vi "Get Fit Length.vi"(8 "error in (no error)":errorcluster, 11 "Abstract Fit in":refnum<class "Abstract Fit.lvclass">) -> (0 "error out":errorcluster, 2 "Length":i32, 3 "Abstract Fit out":refnum<class "Abstract Fit.lvclass">)   [LabVIEW 2016, in "Abstract Fit.lvclass"]
uses:
  Abstract Fit.lvclass
  Abstract Fit.lvclass/Abstract Fit.ctl
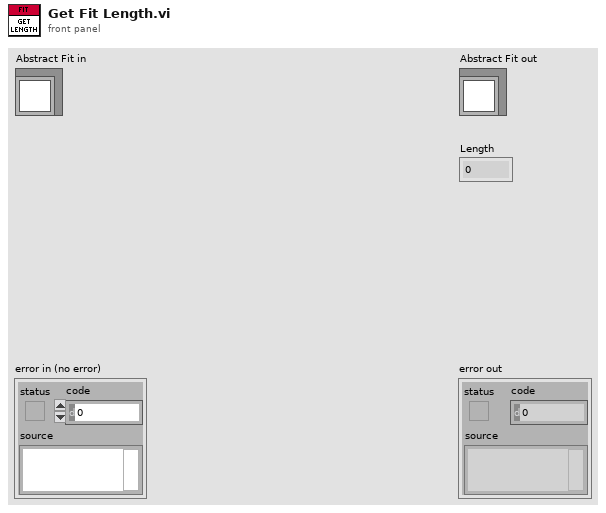
[diagram p1: front panel]
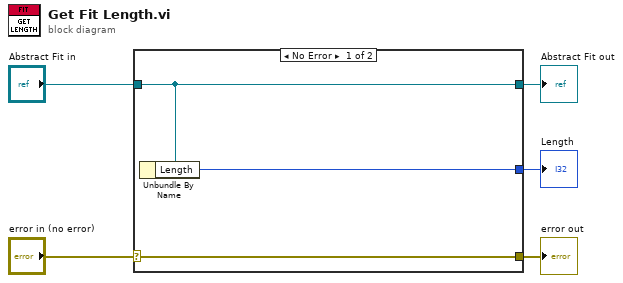
[diagram p0: block diagram]
diagram:
  n1 = case shown="No Error" "error in (no error)" {
    selector: "error in (no error)" -> [w8 w9]
    tunnel: [w8 w9] -> w4
    tunnel: [w7 w10] -> w2
    tunnel: "Abstract Fit in" -> [w7 w10]
    tunnel: [w6 _] -> w1
    frame No Error {
      n2 = Unbundle By Name(w7) -> ("Length"=w6:i32)
    }
    frame Error {
    }
  }
  "error out" <- w4
  "Abstract Fit out" <- w2
  "Length" <- w1
